vi "MGCC_LoadFcst_main.vi"() -> ()   [LabVIEW 2016]
doc: "-----------------------------------------------------------------------------------------------------------------------\nCopyright <2019> <The University of Tennessee at Knoxville and the University of Tennessee Research Foundation>\nThis software is released under BSD-3 \nhttps://opensource.org/licenses/BSD-3-Clause \nAdditional license options available at https://utrf.tennessee.edu/industry/sample-agreements/\n-----------------------------------------------------------------------------------------------------------------------\n\nThis VI implements a load forecasting function for the microgrid. The VI will also use measurements from local controllers to calculate the load as the controller is running. The Sub-VI \"MGCC_LoadFcst.vi\" is called to perform an ARMA regression on historical data and generate forecasts for the next 24-hour period. A universal timer can be easily added to control the triggering of this VI."
uses:
  Finite State Machine/Sub-VIs/MGCC_FntStaMach_gobal.vi
  <vilib>/Utility/error.llb/Error Cluster From Error Code.vi
  Communication/Global communication.vi
  <vilib>/ErrorRing/Error Ring.xnode
  <vilib>/Analysis/NI_AALBase.lvlib
panel:
  out "Forecast":dbl[](graph)
  out "Weekend_History":dbl[](graph)
  out "Weekday_History":dbl[](graph)
  out "err1":errorcluster
  out "f_MGCC_LoadFcst_FcstLoad":dbl[](array[numeric])
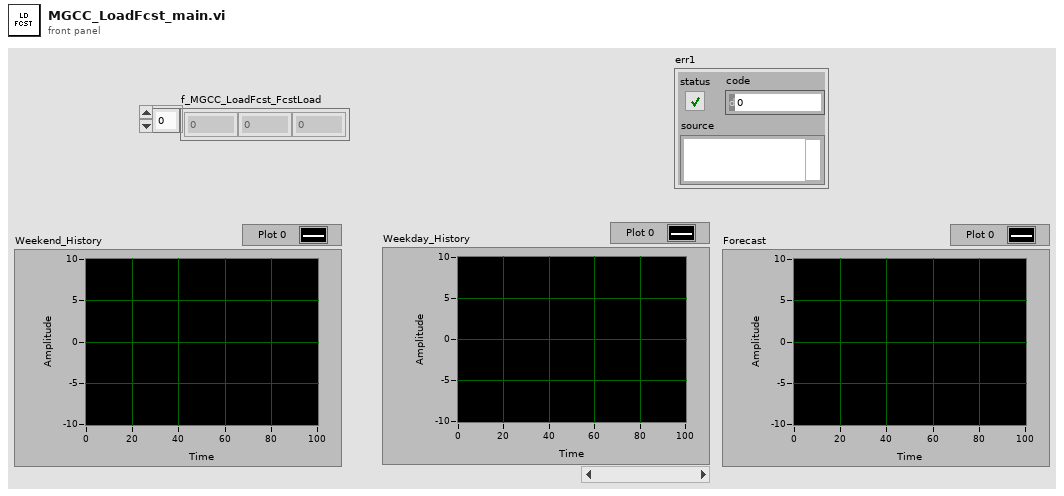
[diagram p1: front panel]
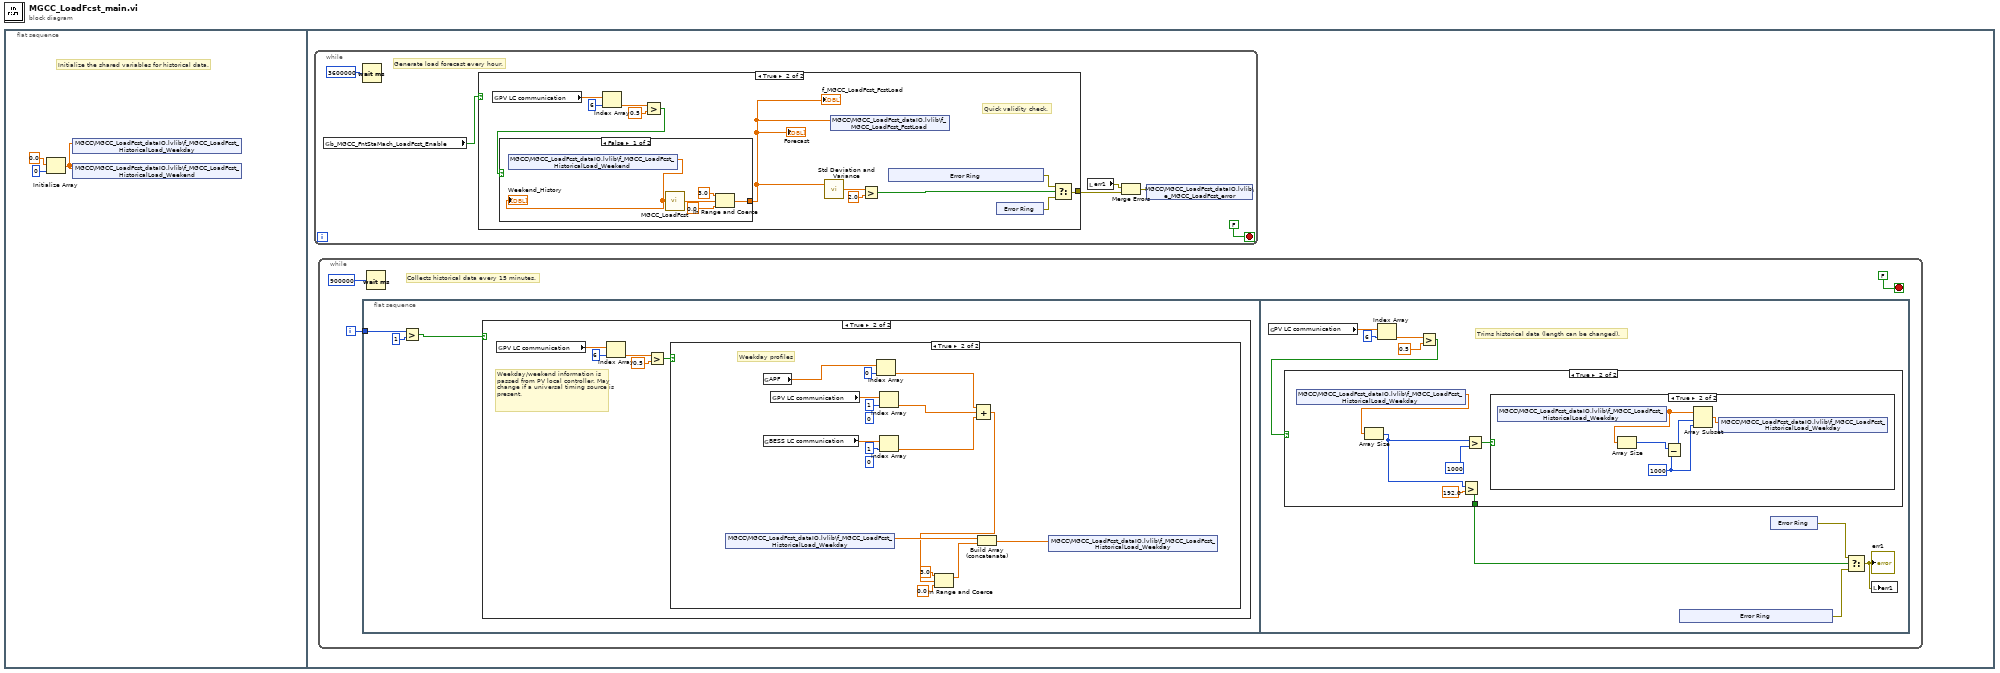
[diagram p0: block diagram]
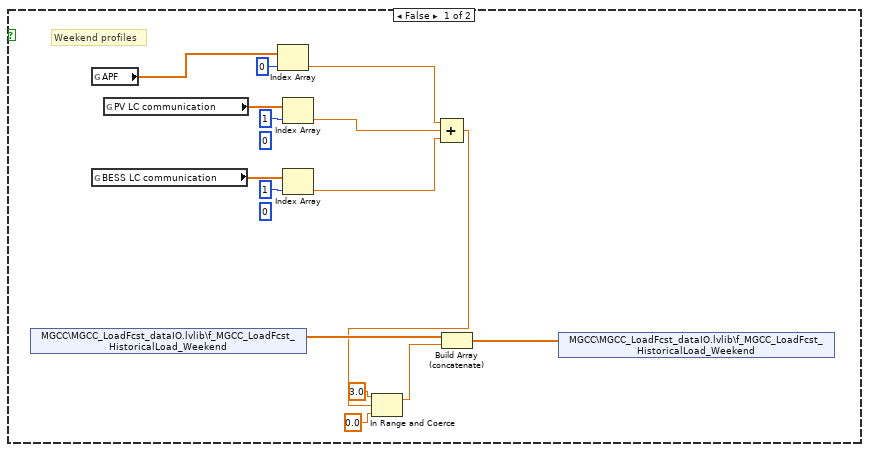
[diagram p3: hidden frame]
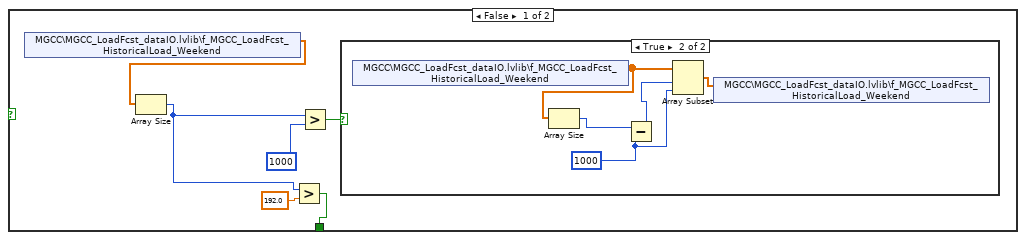
[diagram p4: hidden frame]
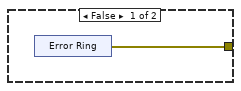
[diagram p7: hidden frame]
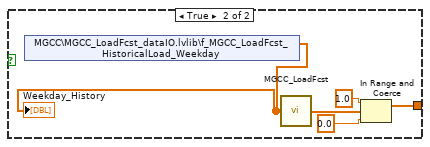
[diagram p8: hidden frame]
diagram:
  n1 = flat-sequence {
    frame #0 {
      # "Initialize the shared variables for historical data."
      n2 = Initialize Array(0.0 ("element"), 0 ("dimension size")) -> (w1:dbl[])
      n3 = shared-variable "MGCC\\MGCC_LoadFcst_dataIO.lvlib\\f_MGCC_LoadFcst_HistoricalLoad_Weekday"(w1) -> ()  [unwired: 1 in, 1 out]
      n4 = shared-variable "MGCC\\MGCC_LoadFcst_dataIO.lvlib\\f_MGCC_LoadFcst_HistoricalLoad_Weekend"(w1) -> ()  [unwired: 1 in, 1 out]
    }
    frame #1 {
      n5 = while {
        stop <- FALSE stop-if-true
        # "Generate load forecast every hour."
        n6 = global read "MGCC_FntStaMach_gobal.vi" "b_MGCC_FntStaMach_LoadFcst_Enable"() -> (w82:bool)
        n7 = Wait (ms)(milliseconds to wait=u32 3600000) -> ()  [unwired: 1 out]
        n8 = case shown="True" w82 {
          tunnel: [w88 w99] -> w85
          frame False {
            n9 = xnode "Error Ring"() -> ("error out"=w88:errorcluster)
          }
          frame True {
            # "Quick validity check."
            n10 = global read "Global communication.vi" "PV LC communication"() -> (w98:dbl[])
            n11 = Index Array(array=w98, index=6) -> (element=w96:dbl)
            n12 = Greater?(x=w96, y=0.5) -> (0:w94:bool)
            n13 = case shown="False" w94 {
              tunnel: [w103 w107] -> w91
              frame False {
                n14 = shared-variable "MGCC\\MGCC_LoadFcst_dataIO.lvlib\\f_MGCC_LoadFcst_HistoricalLoad_Weekend"() -> (w102:dbl[])  [unwired: 1 in, 1 out]
                "Weekend_History" <- w102
                n15 = call "MGCC_LoadFcst.vi"("InputTimeSeries"=w102) -> ("OutputTimeSeries"=w106:dbl[])
                n16 = In Range and Coerce(upper limit=3.0, x=w106, lower limit=0.0) -> (coerced(x)=w103:dbl[])  [unwired: 1 out]
              }
              frame True {
                n17 = shared-variable "MGCC\\MGCC_LoadFcst_dataIO.lvlib\\f_MGCC_LoadFcst_HistoricalLoad_Weekday"() -> (w109:dbl[])  [unwired: 1 in, 1 out]
                "Weekday_History" <- w109
                n18 = call "MGCC_LoadFcst.vi"("InputTimeSeries"=w109) -> ("OutputTimeSeries"=w108:dbl[])
                n19 = In Range and Coerce(upper limit=1.0, x=w108, lower limit=0.0) -> (coerced(x)=w107:dbl[])  [unwired: 1 out]
              }
            }
            "f_MGCC_LoadFcst_FcstLoad" <- w91
            "Forecast" <- w91
            n20 = call <vilib>:"Std Deviation and Variance.vi"("X"=w91) -> ("standard deviation"=w93:dbl)  [unwired: 1 in, 2 out]
            n21 = shared-variable "MGCC\\MGCC_LoadFcst_dataIO.lvlib\\f_MGCC_LoadFcst_FcstLoad"(w91) -> ()  [unwired: 1 in, 1 out]
            n22 = Greater?(x=w93, y=2.0) -> (0:w90:bool)
            n23 = xnode "Error Ring"() -> ("error out"=w100:errorcluster)
            n24 = xnode "Error Ring"() -> ("error out"=w101:errorcluster)
            n25 = Select(t=w100, s=w90, f=w101) -> (s? t:f=w99:errorcluster)
          }
        }
        n26 = local read "err1"() -> (w83:errorcluster)
        n27 = Merge Errors(w83, w85) -> (w84:errorcluster)
        n28 = shared-variable "MGCC\\MGCC_LoadFcst_dataIO.lvlib\\e_MGCC_LoadFcst_error"(w84) -> ()  [unwired: 1 in, 1 out]
      }
      n29 = while {
        i -> [w4]
        stop <- FALSE stop-if-true
        # "Collects historical data every 15 minutes."
        n30 = flat-sequence {
          tunnel: w4 -> [w9]
          frame #0 {
            n31 = Greater?(x=w9, y=1) -> (0:w7:bool)
            n32 = case shown="True" w7 {
              frame False {
              }
              frame True {
                # "Weekday/weekend information is passed from PV local controller. May change if a universal timing source is present."
                n33 = global read "Global communication.vi" "PV LC communication"() -> (w14:dbl[])
                n34 = Index Array(array=w14, index=6) -> (element=w12:dbl)
                n35 = Greater?(x=w12, y=0.5) -> (0:w10:bool)
                n36 = case shown="True" w10 {
                  frame False {
                    (unwired) 0 ("index")
                    (unwired) 0 ("index")
                    # "Weekend profiles"
                    n37 = shared-variable "MGCC\\MGCC_LoadFcst_dataIO.lvlib\\f_MGCC_LoadFcst_HistoricalLoad_Weekend"() -> (w22:dbl[])  [unwired: 1 in, 1 out]
                    n38 = global read "Global communication.vi" "APF"() -> (w21:dbl[])
                    n39 = global read "Global communication.vi" "BESS LC communication"() -> (w28:dbl[])
                    n40 = global read "Global communication.vi" "PV LC communication"() -> (w29:dbl[])
                    n41 = Index Array(array=w21, index=0) -> (element=w19:dbl)
                    n42 = Index Array(array=w29, index=1) -> (element=w18:dbl)
                    n43 = Index Array(array=w28, index=1) -> (element=w17:dbl)
                    n44 = Compound Arithmetic op=ADD(w19, w18, w17) -> (w16:dbl)
                    n45 = In Range and Coerce(upper limit=3.0, x=w16, lower limit=0.0) -> (coerced(x)=w23:dbl)  [unwired: 1 out]
                    n46 = Build Array (concatenate)(w22, w23) -> (w15:dbl[])
                    n47 = shared-variable "MGCC\\MGCC_LoadFcst_dataIO.lvlib\\f_MGCC_LoadFcst_HistoricalLoad_Weekend"(w15) -> ()  [unwired: 1 in, 1 out]
                  }
                  frame True {
                    (unwired) 0 ("index")
                    (unwired) 0 ("index")
                    # "Weekday profiles"
                    n48 = shared-variable "MGCC\\MGCC_LoadFcst_dataIO.lvlib\\f_MGCC_LoadFcst_HistoricalLoad_Weekday"() -> (w37:dbl[])  [unwired: 1 in, 1 out]
                    n49 = global read "Global communication.vi" "APF"() -> (w36:dbl[])
                    n50 = global read "Global communication.vi" "BESS LC communication"() -> (w43:dbl[])
                    n51 = global read "Global communication.vi" "PV LC communication"() -> (w44:dbl[])
                    n52 = Index Array(array=w36, index=0) -> (element=w34:dbl)
                    n53 = Index Array(array=w44, index=1) -> (element=w33:dbl)
                    n54 = Index Array(array=w43, index=1) -> (element=w32:dbl)
                    n55 = Compound Arithmetic op=ADD(w34, w33, w32) -> (w31:dbl)
                    n56 = In Range and Coerce(upper limit=3.0, x=w31, lower limit=0.0) -> (coerced(x)=w38:dbl)  [unwired: 1 out]
                    n57 = Build Array (concatenate)(w37, w38) -> (w30:dbl[])
                    n58 = shared-variable "MGCC\\MGCC_LoadFcst_dataIO.lvlib\\f_MGCC_LoadFcst_HistoricalLoad_Weekday"(w30) -> ()  [unwired: 1 in, 1 out]
                  }
                }
              }
            }
          }
          frame #1 {
            # "Trims historical data (length can be changed)."
            n59 = global read "Global communication.vi" "PV LC communication"() -> (w49:dbl[])
            n60 = Index Array(array=w49, index=6) -> (element=w47:dbl)
            n61 = Greater?(x=w47, y=0.5) -> (0:w45:bool)
            n62 = case shown="True" w45 {
              tunnel: [w55 w67] -> w53
              frame False {
                n63 = shared-variable "MGCC\\MGCC_LoadFcst_dataIO.lvlib\\f_MGCC_LoadFcst_HistoricalLoad_Weekend"() -> (w56:dbl[])  [unwired: 1 in, 1 out]
                n64 = Array Size(array=w56) -> (size(s)=w54:i32)
                n65 = Greater?(x=w54, y=192.0) -> (0:w55:bool)
                n66 = Greater?(x=w54, y=1000) -> (0:w59:bool)
                n67 = case shown="True" w59 {
                  frame False {
                  }
                  frame True {
                    w60 = 1000 ("y")
                    n68 = shared-variable "MGCC\\MGCC_LoadFcst_dataIO.lvlib\\f_MGCC_LoadFcst_HistoricalLoad_Weekend"() -> (w64:dbl[])  [unwired: 1 in, 1 out]
                    n69 = Array Size(array=w64) -> (size(s)=w62:i32)
                    n70 = Subtract(x=w62, y=w60) -> (x-y=w61:i32)
                    n71 = Array Subset(array=w64, index=w61, length=w60) -> (w63:dbl[])
                    n72 = shared-variable "MGCC\\MGCC_LoadFcst_dataIO.lvlib\\f_MGCC_LoadFcst_HistoricalLoad_Weekend"(w63) -> ()  [unwired: 1 in, 1 out]
                  }
                }
              }
              frame True {
                n73 = shared-variable "MGCC\\MGCC_LoadFcst_dataIO.lvlib\\f_MGCC_LoadFcst_HistoricalLoad_Weekday"() -> (w66:dbl[])  [unwired: 1 in, 1 out]
                n74 = Array Size(array=w66) -> (size(s)=w65:i32)
                n75 = Greater?(x=w65, y=192.0) -> (0:w67:bool)
                n76 = Greater?(x=w65, y=1000) -> (0:w70:bool)
                n77 = case shown="True" w70 {
                  frame False {
                  }
                  frame True {
                    w72 = 1000 ("y")
                    n78 = shared-variable "MGCC\\MGCC_LoadFcst_dataIO.lvlib\\f_MGCC_LoadFcst_HistoricalLoad_Weekday"() -> (w75:dbl[])  [unwired: 1 in, 1 out]
                    n79 = Array Size(array=w75) -> (size(s)=w73:i32)
                    n80 = Subtract(x=w73, y=w72) -> (x-y=w71:i32)
                    n81 = Array Subset(array=w75, index=w71, length=w72) -> (w74:dbl[])
                    n82 = shared-variable "MGCC\\MGCC_LoadFcst_dataIO.lvlib\\f_MGCC_LoadFcst_HistoricalLoad_Weekday"(w74) -> ()  [unwired: 1 in, 1 out]
                  }
                }
              }
            }
            n83 = xnode "Error Ring"() -> ("error out"=w51:errorcluster)
            n84 = xnode "Error Ring"() -> ("error out"=w52:errorcluster)
            n85 = Select(t=w52, s=w53, f=w51) -> (s? t:f=w50:errorcluster)
            "err1" <- w50
            n86 = local write "err1"(w50) -> ()
          }
        }
        n87 = Wait (ms)(milliseconds to wait=u32 900000) -> ()  [unwired: 1 out]
      }
    }
  }
